vi "ADS Type ID to .NET Type.vi"(8 "error in (no error)":errorcluster, 9 "Type ID":i32(ring) items=["ADST_VOID"=0, "ADST_INT16"=2, "ADST_INT32"=3, "ADST_REAL32"=4, "ADST_REAL64"=5, "ADST_INT8"=16, "ADST_UINT8"=17, "ADST_UINT16"=18, "ADST_UINT32"=19, "ADST_INT64"=20, "ADST_UINT64"=21, "ADST_STRING"=30, "ADST_WSTRING"=31, "ADST_REAL80"=32, "ADST_BIT"=33, "ADST_MAXTYPES"=34, "ADST_BIGTYPE"=65], 11 "TwinCAT ADS in":refnum<class "TwinCAT ADS.lvclass">) -> (0 "error out":errorcluster, 1 ".NET Type":refnum<k24>, 3 "TwinCAT ADS out":refnum<class "TwinCAT ADS.lvclass">)   [LabVIEW 2018, in "TwinCAT ADS.lvclass"]
uses:
  TwinCAT ADS.lvclass
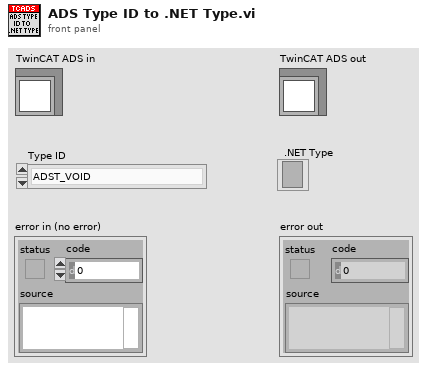
[diagram p1: front panel]
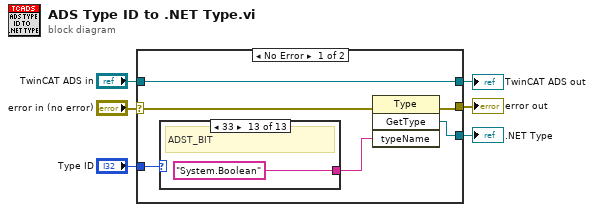
[diagram p0: block diagram]
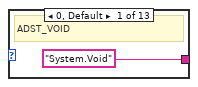
[diagram p2: hidden frame]
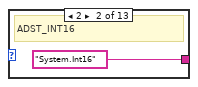
[diagram p3: hidden frame]
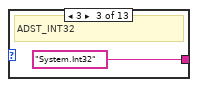
[diagram p4: hidden frame]
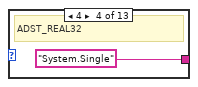
[diagram p5: hidden frame]
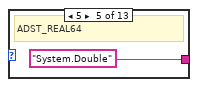
[diagram p6: hidden frame]
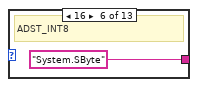
[diagram p7: hidden frame]
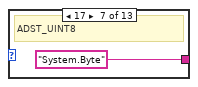
[diagram p8: hidden frame]
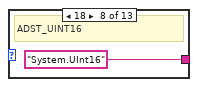
[diagram p9: hidden frame]
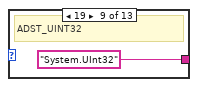
[diagram p10: hidden frame]
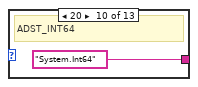
[diagram p11: hidden frame]
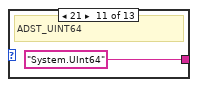
[diagram p12: hidden frame]
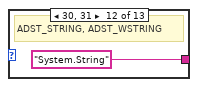
[diagram p13: hidden frame]
diagram:
  n1 = case shown="No Error" "error in (no error)" {
    selector: "error in (no error)" -> [w9 w27]
    tunnel: [w8 w27] -> w5
    tunnel: [w12 w26] -> w3
    tunnel: "TwinCAT ADS in" -> [w12 w26]
    tunnel: "Type ID" -> [w11 _]
    tunnel: [w7 _] -> w1
    frame No Error {
      n2 = case shown="33" w11 {
        tunnel: ["System.Void" ("typeName") "System.Int16" ("typeName") "System.Int32" ("typeName") "System.Single" ("typeName") "System.Double" ("typeName") "System.SByte" ("typeName") "System.Byte" ("typeName") "System.UInt16" ("typeName") "System.UInt32" ("typeName") "System.Int64" ("typeName") "System.UInt64" ("typeName") "System.String" ("typeName") "System.Boolean" ("typeName")] -> w10
        frame 0, Default {
          # "ADST_VOID"
        }
        frame 2 {
          # "ADST_INT16"
        }
        frame 3 {
          # "ADST_INT32"
        }
        frame 4 {
          # "ADST_REAL32"
        }
        frame 5 {
          # "ADST_REAL64"
        }
        frame 16 {
          # "ADST_INT8"
        }
        frame 17 {
          # "ADST_UINT8"
        }
        frame 18 {
          # "ADST_UINT16"
        }
        frame 19 {
          # "ADST_UINT32"
        }
        frame 20 {
          # "ADST_INT64"
        }
        frame 21 {
          # "ADST_UINT64"
        }
        frame 30, 31 {
          # "ADST_STRING, ADST_WSTRING"
        }
        frame 33 {
          # "ADST_BIT"
        }
      }
      n3 = invoke class="Type" method="GetType"(error in=w9, "typeName"=w10) -> (error out=w8:errorcluster, "GetType"=w7:refnum<k24>)  [unwired: 2 in, 2 out]
    }
    frame Error {
    }
  }
  "error out" <- w5
  "TwinCAT ADS out" <- w3
  ".NET Type" <- w1
